vi "Build Generic Socket CAN.vi"(7 "extended?":bool=TRUE, 8 "Interface Mode":T1(ring)=enum."CAN FD BRS", 9 "Payload":u8[](array[numeric])=[10, 11, 10, 13, 11, 10, 11, 14] format="%.0x", 10 "identifier":u32=9 format="%.0x", 11 "pcap Parse and Build in":refnum<class "pcap Parse and Build.lvclass">) -> (2 "CAN Packet":u8[](array[numeric]), 3 "pcap Parse and Build out":refnum<class "pcap Parse and Build.lvclass">)   [LabVIEW 2021, in "pcap Parse and Build.lvclass"]
uses:
  pcap Parse and Build.lvclass
  Typedef/Socket CAN Header.ctl
  pcap Parse and Build.lvclass/pcap Parse and Build.ctl
  <vilib>/CIF Foundation/CIF Utilities/Time/System Time/LabVIEW Time to TAI Time.vi
  Build/SubVIs/Flatten SocketCAN Header.vi/e4177ba7-55c0-4140-bea2-15e5e44a53d0.vi
  Build/SubVIs/Flatten Packet Header.vi
  Build/SubVIs/Flatten SocketCAN Header.vi/e4177ba7-55c0-4140-bea2-15e5e44a53d0.vi/c28b0ead-42ad-4072-80a2-aca7f2bd7ce3.vi
  Build/SubVIs/Flatten Packet Header.vi/e4177ba7-55c0-4140-bea2-15e5e44a53d0.vi
  Build/SubVIs/Flatten Packet Header.vi/e4177ba7-55c0-4140-bea2-15e5e44a53d0.vi/c28b0ead-42ad-4072-80a2-aca7f2bd7ce3.vi
  <vilib>/CIF Foundation/CIF Utilities/Time/Time_CIF_U.lvlib
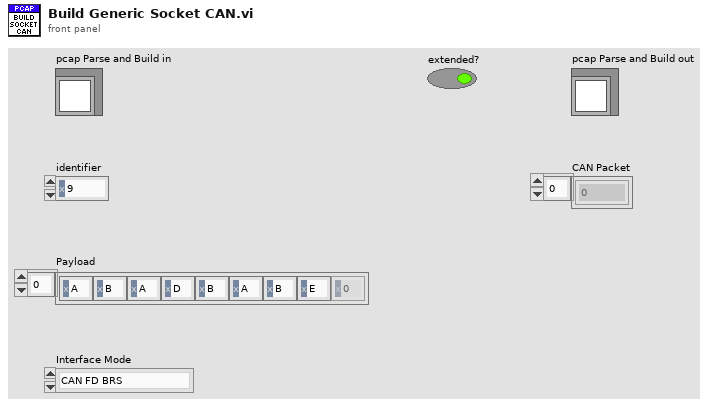
[diagram p1: front panel]
types:
  T1 = enum16{"CAN 2.0", "CAN FD", "CAN FD BRS", "Remote"}
  T2 = typedef "pcap Parse and Build.lvclass/Socket CAN Header.ctl" = cluster{"CANID and Flags":u32, "Payload Length":u8, "FD Flags":u8, "RSVD":u8, "Len8 DLC":u8}
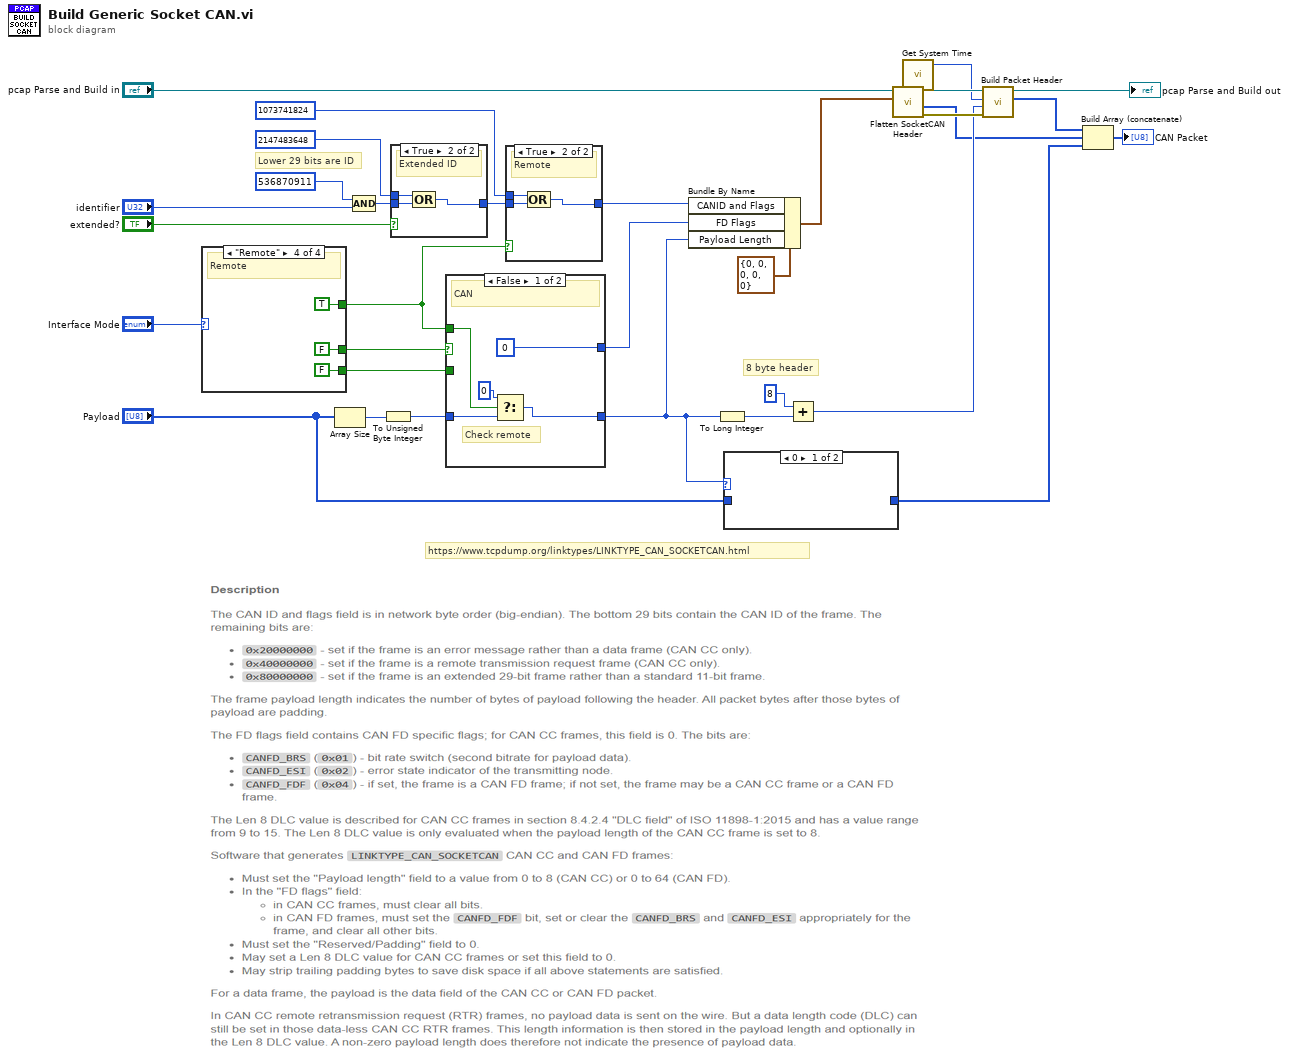
[diagram p0: block diagram]
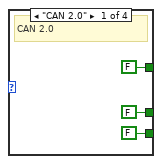
[diagram p3: hidden frame]
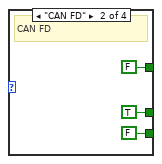
[diagram p4: hidden frame]
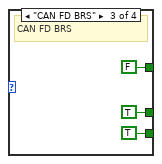
[diagram p5: hidden frame]
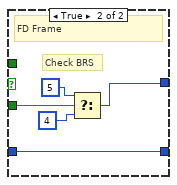
[diagram p8: hidden frame]
diagram:
  # "8 byte header"
  # "Lower 29 bits are ID"
  # "https://www.tcpdump.org/linktypes/LINKTYPE_CAN_SOCKETCAN.html"
  n1 = case shown="\"Remote\"" "Interface Mode" {
    tunnel: [FALSE FALSE FALSE TRUE] -> w19
    tunnel: [FALSE TRUE TRUE FALSE] -> w16
    tunnel: [FALSE FALSE TRUE FALSE] -> w17
    frame "CAN 2.0" {
      # "CAN 2.0"
    }
    frame "CAN FD" {
      # "CAN FD"
    }
    frame "CAN FD BRS" {
      # "CAN FD BRS"
    }
    frame "Remote" {
      # "Remote"
    }
  }
  n2 = Array Size(array="Payload") -> (size(s)=w20:i32)
  n3 = Compound Arithmetic op=AND(u32 536870911 ("number"), "identifier") -> (w26:u32)
  n4 = To Unsigned Byte Integer(number=w20) -> (unsigned 8bit integer=w18:u8)
  n5 = case shown="True" "extended?" {
    tunnel: w26 -> [w44 w47]
    tunnel: u32 2147483648 -> [_ w46]
    tunnel: [w44 w45] -> w24
    frame False {
    }
    frame True {
      # "Extended ID"
      n6 = Compound Arithmetic op=OR(w46, w47) -> (w45:u32)
    }
  }
  n7 = case shown="False" w16 {
    tunnel: w17 -> [_ w56]
    tunnel: [u8 0 w53] -> w21
    tunnel: w18 -> [w51 w57]
    tunnel: [w48 w57] -> w6
    tunnel: w19 -> [w50 _]
    frame False {
      # "Check remote"
      # "CAN"
      n8 = Select(t=u8 0, s=w50, f=w51) -> (s? t:f=w48:u8)
    }
    frame True {
      # "Check BRS"
      # "FD Frame"
      n9 = Select(t=u8 5, s=w56, f=u8 4) -> (s? t:f=w53:u8)
    }
  }
  n10 = case shown="True" w19 {
    tunnel: w24 -> [w58 w61]
    tunnel: [w58 w60] -> w22
    tunnel: u32 1073741824 -> [_ w59]
    frame False {
    }
    frame True {
      # "Remote"
      n11 = Compound Arithmetic op=OR(w59, w61) -> (w60:u32)
    }
  }
  n12 = Bundle By Name(cluster=T2 {"CANID and Flags"=0, "Payload Length"=0, "FD Flags"=0, "RSVD"=0, "Len8 DLC"=0} ("CAN Header out 2"), "CANID and Flags"=w22, "FD Flags"=w21, "Payload Length"=w6) -> (w9:T2)
  n13 = To Long Integer(number=w6) -> (32bit integer=w14:i32)
  n14 = case shown="0" w6 {
    tunnel: "Payload" -> [_ w62]
    tunnel: [_ w62] -> w4
    frame 0 {
    }
    frame 1, Default {
    }
  }
  n15 = Add(x=8, y=w14) -> (x+y=w8:i32)
  n16 = call "Flatten SocketCAN Header.vi"("CAN Header in"=w9, "pcap Parse and Build in"="pcap Parse and Build in") -> ("error out"=w28:errorcluster, "Flattened Data out"=w2:u8[], "pcap Parse and Build out"=w29:refnum<class "pcap Parse and Build.lvclass">)  [unwired: 6 in, 1 out]
  n17 = call <vilib>:"Get System Time.vi"() -> ("Time (ns)"=w7:i64)  [unwired: 5 in]
  n18 = call "Build Packet Header.vi"("error in (no error)"=w28, "Length"=w8, "TAI Time (ns)"=w7, "pcap Parse and Build in"=w29) -> ("Flattened Data out"=w3:u8[], "pcap Parse and Build out"=→"pcap Parse and Build out":refnum<class "pcap Parse and Build.lvclass">)  [unwired: 5 in, 1 out]
  n19 = Build Array (concatenate)(w3, w2, w4) -> (→"CAN Packet":u8[])
